vi "AlliGator Source Image Profile Window.vi"() -> ()   [LabVIEW 2021, in "AlliGator Image Profile Window.lvlib"]
doc: "AlliGator Profile Window."
uses:
  AlliGator Image Profile Window.lvlib
  Globals, Variables, Constants/AlliGator Variables List.ctl
  Action Engine/AlliGator Q Element.ctl
  Action Engine/AlliGator Q Event.ctl
  AlliGator Image Profile Data.ctl
  Image/Image ROI Type.ctl
  AlliGator Image Profile Plot Data.ctl
  Graphs/XY Graph/XY Plot Data.ctl
  Graphs/XY Graph/XY Graph Event.ctl
  <vilib>/Utility/miscctls.llb/LVPoint32TypeDef.ctl
  Image/Box Profile Type.ctl
  Graphs/XY Graph/XY Graph Add-Ons.lvlib
  Globals, Variables, Constants/AlliGator Globals, Variables & Constants.lvlib
  Notebook/Notebook.lvlib
  Rich Text Box/Rich Text Box.lvlib
  Settings/AlliGator Settings.lvlib
  Image/Image.lvlib
  Action Engine/AlliGator Action Engine.lvlib
  Error/Error.lvlib
panel:
  out "Image Profile TipStrip":string
  out "Image Profile":cluster{"X Array":dbl[], "Y Array":dbl[]}[](graph) caption="No Selection Profile (0,0)-(0,0)"
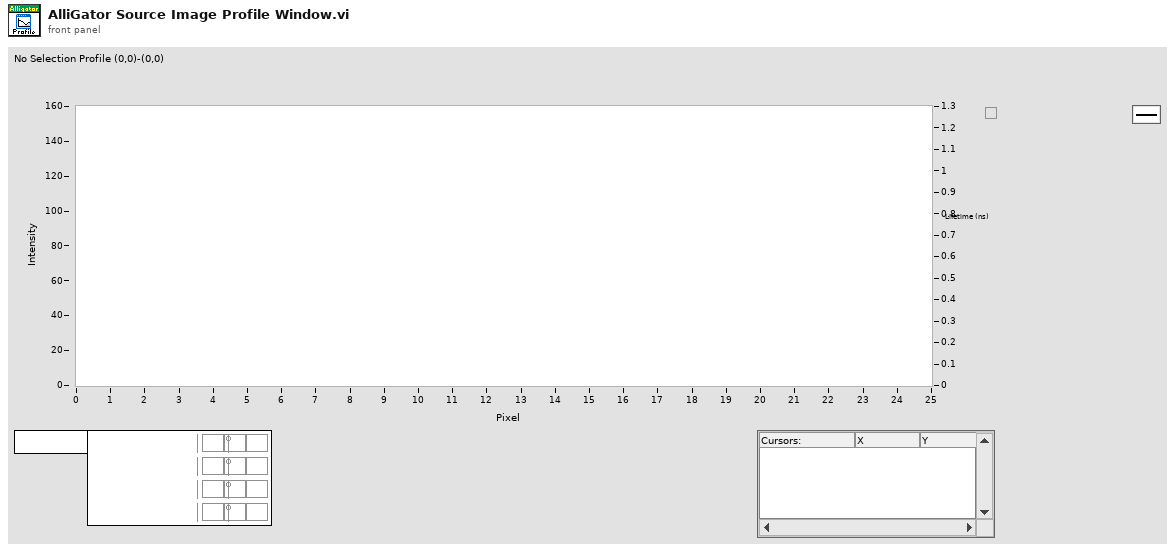
[diagram p1: front panel]
types:
  T1 = typedef "AlliGator Action Engine.lvlib/AlliGator Q Element.ctl" = cluster{"AlliGator Q Event":T2, "Data":variant}
  T2 = typedef "AlliGator Action Engine.lvlib/AlliGator Q Event.ctl" = enum16{"---- Files ----", "Files:Set Batch Export Files To Save", "Files:Set Dataset Loading & Pre-processing Options", "Files:Check #Frames in Dataset", "Files:Increment Frame Index", "Files:Open Mask Image", "Files:Open White Light Image", "Files:Open Single Dataset", "Files:New Folder of Folders Selected", "Files:Load File (all Types)_Scriptable", "Files:Move Flattened Series to Folders Series", "Files:Select Folder", "Files:Load FLI Dataset", "Files:Load Swiss SPAD 1 Dataset", "Files:Load Swiss SPAD 2 Dataset", "Files:Load .sdt FLI Dataset", "Files:Load .ptu FLI Dataset", "Files:Load .bin FLI Dataset", "Files:Load Single Gate Image Folder", "Files:Load I/m/phi Dataset (deprecated)", "Files:Load Single Image", "Files:Subtract Background File", "Files:Export FLI Dataset", "Files:Load HDF5 FLI Dataset", "Files:Set Destination File Path", "Files:Save Mask Image", "Files:Batch Conversion", "Files:New Folder Selected", "Files:Close FLI Dataset", "Files:Close FLI Dataset Series", "Files:Close White Light Image", "Files:Close Mask Image", "---- FLI Dataset ----", "FLI Dataset:Channel Arithmetic", "FLI Dataset:Export Average Lifetime Map as ASCII", "FLI Dataset:Export User-Defined Quantity Map as ASCII", "FLI Dataset:Python Function FLI Dataset Event", "FLI Dataset:ROI Analysis", "FLI Dataset:Tilted Logistic Square Gated IRF Characteristics Map", "FLI Dataset:Logistic Square Gated IRF Characteristics Map", "FLI Dataset:Square Gated IRF Characteristics Map", "FLI Dataset:Multi-ROI Single-Pixel Phasor Analysis", "FLI Dataset:Multi-ROI Single-Pixel NLSF Analysis", "FLI Dataset:All ROIs IRF Extraction", "FLI Dataset:All ROIs Decay Fit Non-Interactive (Fast + Individual IRF)", "FLI Dataset:All ROIs Phasor Analysis", "FLI Dataset:All ROIs Decay Fit", "FLI Dataset:Fluorescence Decay Statistics", "FLI Dataset:Update Decay Statistics Graph", "FLI Dataset:Get Decay from ROI", "FLI Dataset:All ROIs Average Lifetimes", "FLI Dataset:Save/Load Local IRFs", "FLI Dataset:Clear Local IRFs", "---- FLI Dataset Series ----", "FLI Dataset Series:Sum All Datasets in Series", "FLI Dataset Series:Add Dataset to Accumulated Dataset", "FLI Dataset Series:Display Accumulated Dataset", "FLI Dataset Series:Clear Dataset Series Sum", "FLI Dataset Series:Time-Series Analysis (NLSF)", "FLI Dataset Series:Time-Series Analysis (Phasor)", "---- Image ----", "Image:Update Image Profile Plots", "Image:Image Histogram Cursor Move", "Image:Image Histogram", "Image:Image Contrast", "Image:Set Image Histogram Cursor Move Flag", "Image:Clear Image Overlay", "Image:Use ROI as Search Area", "Image:Set ROI Diameter", "Image:Save Image Data as TIFF", "Image:Save Displayed Image with Overlay", "Image:Save Image Overlay Only", "Image:Save Image as Hot Pixel Mask", "Image:Change Source Image Color Palette", "Image:Copy Image to Clipboard", "Image:Source Image ROI Selection", "Image:Delete All ROIs", "Image:Delete All Unselected ROIs", "Image:Delete ROI", "Image:Merge All ROIs", "Image:Store ROI", "Image:Source Image ROI Storage", "Image:Export ROI Description to Notebook", "Image:Save ROI", "Image:Load ROI", "Image:Paste ROI Definition", "Image:Clear ROI", "Image:Identify ROIs in Mask Image", "Image:Create Complementary ROI", "Image:Create Contour ROI", "Image:Create ROI(s) from Pixels with Peak above Min_Scriptable", "Image:Create ROI(s) from Pixels with Intensity above Min_Scriptable", "Image:Compute ROI Statistics", "Image:Delete ROI(s) based on ROI Characteristics", "Image:Create ROI Grid", "Image:ROI to Individual Pixel ROIs", "Image:Python Function Source Image Event", "Image:Show Phasor Calibration Map ROI Centers", "Image:Convert ROI to Mask Image", "Image:Mouse Move", "Image:Mouse Up", "Image:Set Source Image Mouse Move Flag", "Image:Add Scale Bar Overlay", "Image:Delete Existing ROIs Option", "Image:Overlay ROI Median", "Image:Check Current ROI", "---- Decay ----", "Decay:Clear IRF/Reference Plot", "Decay:Add Decay to Graph", "Decay:Smoothen Plot", "Decay:Smoothen Plot Tail", "Decay:Average Selected Plots", "Decay:Extract IRF", "Decay:Optimal IRF Extraction", "Decay:Threshold IRF", "Decay:Fit to Model IRF", "Decay:Fit IRF to Square Gate", "Decay:Fit IRF to Logistic Square Gate", "Decay:Fit IRF to Tilted Logistic Square Gate", "Decay:Create Bounding Cursors Set", "Decay:Export Bounding Cursors Definition to Notebook", "Decay:Denoise Plot", "Decay:Compute Cumulative Function", "Decay:Use as Reference Decay", "Decay:Show Reference Decay/IRF", "Decay:Extrapolate Decay", "Decay:Create Head & Tail Bounding Cursors", "Decay:Store Cursor-defined Head & Tail Fractions", "Decay:Rebin Plot", "Decay:1-Normalize Decay", "Decay:[0-1]-Normalize Plot", "Decay:Straighten Decay", "Decay:Shift Decay", "Decay:Fold Decay", "Decay:Fit Decay", "Decay:Global Fit of Selected Decays", "Decay:Post Global Fit Script", "Decay:Add Global Fit Parameters to Graph", "Decay:Add Decay Parameter(s) to Plot (Graph)", "Decay:Export Decay to Phasor Graph", "Decay:Plot Decay Shifts", "Decay:Compute Average Lifetime", "Decay:Plot Convolution", "Decay:Graph Tip Strip Update", "---- Decay Statistics ----", "Decay Statistics:Tip Strip Update", "---- Intensity Time Trace ----", "Intensity Time Trace:Use File Timestamp", "Intensity Time Trace:Load Intensity Corrections File", "Intensity Time Trace:Clear Intensity Corrections File", "Intensity Time Trace:Tip Strip Update", "---- Phasor Plot ----", "Phasor Plot:Build Phasor Plot", "Phasor Plot:Change Phasor Plot Color Palette", "Phasor Plot:Adjust Phasor Plot Display Range", "Phasor Plot:Highlight Image ROI in Phasor Plot", "Phasor Plot:Save Phasor Plot Image with Overlay", "Phasor Plot:Export Complex Phasor Map", "Phasor Plot:Export Phasor Ratio Map", "Phasor Plot:Export Average Lifetime Map", "Phasor Plot:Compute Phase Lifetime Histogram", "Phasor Plot:Compute Phasor Ratio Histogram", "Phasor Plot:Compute Phase Lifetime vs Intensity Scatter Plot", "Phasor Plot:Weber 2-Component Decomposition", "Phasor Plot:Update Phasor Color Map Vertices", "Phasor Plot:Clear Phasor Overlay", "Phasor Plot:Use Segment Extremities as References", "Phasor Plot:Use UC/Segment Intersections as References", "Phasor Plot:Use UC/Principal Axis Intersections as References", "Phasor Plot:Use UC/Linear Fit Intersections as References", "Phasor Plot:Update Phasor Plot Reference", "Phasor Plot:Show Local Phasor Info in Phasor Plot", "Phasor Plot:Update Phasor Plot State", "Phasor Plot:Phasor Plot ROI Storage", "Phasor Plot:Phasor Plot ROI Selection", "Phasor Plot:Python Function Phasor Plot Event", "Phasor Plot:Overlay Phasor ROI, Ratio or Map in Source Image", "Phasor Plot:Compute Decay of Selected Phasors", "Phasor Plot:Phasor at Image Pixel", "Phasor Plot:Mouse Move", "Phasor Plot:Mouse Up", "Phasor Plot:Display Range Mouse Move", "Phasor Plot:Set Mouse Move Flag", "---- Phasor Graph ----", "Phasor Graph:Calibrated Phasor Map Series", "Phasor Graph:Whole Image Phasor Scatter Plot (deprecated)", "Phasor Graph:Get Phasor Value", "Phasor Graph:Create New Phasor Plot Dialog", "Phasor Graph:Update Last Phasor Value", "Phasor Graph:Update Phasor (m, phi)", "Phasor Graph:Remove Single Phasor from Plot", "Phasor Graph:Add Single Phasor to Plot", "Phasor Graph:Remove Phasor Plot", "Phasor Graph:Remove Selected Phasor Plots", "Phasor Graph:Clear Phasor Data", "Phasor Graph:Clear Phasor Graph", "Phasor Graph:Cursor Move", "Phasor Graph:Draw Cursor Connecting Line", "Phasor Graph:Clear Cursor Connecting Line", "Phasor Graph:Find UC Intersection", "Phasor Graph:Use UC/Cursor-Defined Line Intersections", "Phasor Graph:Use Selected Plots Fitted Line/UC Intersections", "Phasor Graph:Use Selected Plots Principal Axis/UC Intersections", "Phasor Graph:Show Single Phasor", "Phasor Graph:Save Single Phasor Plot", "Phasor Graph:Save All Phasor Plots", "Phasor Graph:Load Phasor Plot(s)", "Phasor Graph:Phasor Multiplication", "Phasor Graph:Compute Average Phasor", "Phasor Graph:Compute Multiple Average Phasors (Selected Plots)", "Phasor Graph:Export Single Phasor Plot Phase Lifetimes", "Phasor Graph:Phase Lifetime Trajectory (deprecated)", "Phasor Graph:Phase Lifetime vs Intensity Scatter Plot (deprecated)", "Phasor Graph:Parameter 2 vs Parameter 1 Scatter Plot", "Phasor Graph:Use Cursor n Location", "Phasor Graph:Set Reference n to Current Phase Lifetime Value", "Phasor Graph:Set Reference n to Lifetime Value", "Phasor Graph:Set Cursor n Location", "Phasor Graph:Save Phasor Graph Image", "Phasor Graph:Update SEPL Plot", "Phasor Graph:Export Single Phasor Plot Data", "Phasor Graph:Export Selected Phasor Plots Data", "Phasor Graph:Python Function Phasor Graph Event", "Phasor Graph:Tip Strip Update", "---- Calibration ----", "Calibration:Set Calibration Type", "Calibration:Load/Save Phasor Calibration", "Calibration:Load/Save Phasor Calibration Series", "Calibration:Load/Save Phasor Calibration Map", "Calibration:Use as Calibration", "Calibration:Compute Optimal Calibration from Phasor References", "Calibration:Clear Phasor Calibration", "Calibration:Single Phasor Calibration Information", "Calibration:Use as Calibration Series", "Calibration:Use as Calibration Map", "Calibration:Clear Calibration Series", "Calibration:Phasor Calibration Series Information", "Calibration:Clear Calibration Map", "Calibration:Phasor Calibration Map Information", "Calibration:Apply Phasor Calibration", "Calibration:Update Single Plot Calibration", "Calibration:Update Multiple Plots Calibration", "Calibration:Clear Single Plot Calibration", "Calibration:Clear All Plots Calibrations", "Calibration:Clear Plot(s) Calibration(s)?", "Calibration:Phasor Calibration Maps (# Gates Series)", "---- Phasor Ratio ----", "Phasor Ratio:Clear Reference n", "Phasor Ratio:Toggle Selected Plot(s)  Lock to Reference 1", "Phasor Ratio:Use as Reference n", "Phasor Ratio:Send Reference n to Notebook", "Phasor Ratio:Toggle Selected Plot(s)  Lock to Reference 2", "Phasor Ratio:Compute Phasor Ratio at Mouse Location", "Phasor Ratio:Compute Phasor Plot's Average Phasor Ratio", "Phasor Ratio:Compute Time-Series Phasor Ratios", "Phasor Ratio:Fit Line to Phasor Ratio Plot", "Phasor Ratio:Save References", "Phasor Ratio:Load References", "Phasor Ratio:Update Phasor Reference 1", "Phasor Ratio:Update Phasor Reference 2", "Phasor Ratio:Move Cursor n to Reference n", "Phasor Ratio:Use as Phasor Reference 1 Lifetime", "Phasor Ratio:Use as Phasor Reference 2 Lifetime", "Phasor Ratio:Export Phasor Ratio Map as ASCII", "Phasor Ratio:Tip Strip Update", "---- Lifetime & Other Parameters Graph ----", "Lifetime:Power Law from Intensity Distribution", "---- Decay Fit Parameter Map ----", "Decay Fit Parameter Map:Export ROI NLSF Data as ASCII", "Decay Fit Parameter Map:Set Decay Fit Parameter Map Selection", "Decay Fit Parameter Map:Build Decay Fit Parameter Map", "Decay Fit Parameter Map:Change Decay Fit Parameter Map Color Palette", "Decay Fit Parameter Map:Export Decay Fit Parameter Map Data as ASCII", "Decay Fit Parameter Map:Export All Decay Fit Parameter Maps Data as ASCII", "Decay Fit Parameter Map:Selected Parameter Scatterplot", "Decay Fit Parameter Map:Parameter 2 vs Parameter 1 Scatterplot", "Decay Fit Parameter Map:Save Decay Fit Parameter Map Image", "Decay Fit Parameter Map:Save-Load IRFs & Fit Data", "Decay Fit Parameter Map:Update Local Decay Plots", "Decay Fit Parameter Map:Python Function Decay Fit Parameters Map Event", "Decay Fit Parameter Map:Overlay Decay Fit Parameter Map in Source Image", "Decay Fit Parameter Map:Selected Parameter vs Intensity Scatterplot", "Decay Fit Parameter Map:Mouse Up", "Decay Fit Parameter Map:Display Range Mouse Move", "Decay Fit Parameter Map:Change Map Resolution", "---- Parameter Map ----", "Parameter Map:Export ROI Parameters Data as ASCII", "Parameter Map:Delete Parameter Map Set", "Parameter Map:Update Parameter List", "Parameter Map:Build Parameter Map", "Parameter Map:Change Parameter Map Color Palette", "Parameter Map:Export Parameter Map Data as ASCII", "Parameter Map:Export All Parameter Maps Data as ASCII", "Parameter Map:Selected Parameter Scatterplot", "Parameter Map:Parameter 2 vs Parameter 1 Scatterplot", "Parameter Map:Selected Parameter vs Intensity Scatterplot", "Parameter Map:Save Parameter Map Image", "Parameter Map:Save-Load IRFs & Parameter Maps (TODO)", "Parameter Map:Set Parameter Map Selection", "Parameter Map:Python Function Parameter Map Event", "Parameter Map:Overlay Parameter Map in Source Image", "Parameter Map:Update Local Decay Plots", "Parameter Map:Mouse Up", "Parameter Map:Display Range Mouse Move", "---- Generic Graph ----", "Generic Graph:Generic XY Graph Event", "Generic Graph:Python Function XY Graph Event", "Generic Graph:New Plot", "Generic Graph:Save Plot", "Generic Graph:XY Plot Histogram", "Generic Graph:Set XY Graph Plot Name", "Generic Graph:Set Last Cursor Style", "Generic Graph:Tip Strip Update", "---- GUI ----", "GUI:Start Script", "GUI:Type of Displayed Image Changed", "GUI:Gate Image Slide Changed", "GUI:Show Busy Icon", "GUI:Show Busy Icon & Abort Button", "GUI:Hide Busy Icon", "GUI:Hide Busy Icon & Abort Button", "GUI:Abort", "GUI:End Script", "GUI:Start Timing", "GUI:End Timing", "GUI:Set State Indicator", "GUI:Send Parameters JSON Strings to Clipboard", "GUI:Set Gate Step", "GUI:Idle", "GUI:Initialization", "GUI:Quit", "GUI:Increment Dataset Index", "GUI:Set Dataset Index to -1", "GUI:Time Series Slider Moved", "GUI:Time Series Slider Changed", "GUI:Toggle Playback or Loop", "GUI:Playback Script", "GUI:Set Phasor Frequency", "GUI:Open Window", "GUI:Start Test Script", "GUI:End Test Script", "DEBUG"}
  T3 = typedef "AlliGator Globals, Variables & Constants.lvlib/AlliGator Variables List.ctl" = enum16{"---- GUI ----", "GUI:Initialization Status", "GUI:State Indicators Refnum", "GUI:Original AlliGator Menu Items", "GUI:Current Action Loop State", "GUI:Script in progress", "GUI:Playback", "GUI:Loop Playback", "GUI:Search ROI Used", "GUI:Search ROI", "Decay Graph Max Legend Size", "Intensity Graph Max Legend Size", "Decay Statistics Graph Max Legend Size", "Phasor Graph Max Legend Size", "Phasor Ratio Graph Max Legend Size", "Lifetime Graph Max Legend Size", "---- Files ----", "Files:Export Dataset Frames as Individual Files", "Files:Show Batch Export Help Balloons", "Files:Frames in Dataset", "Files:ptu File Frame Start Indices", "Files:Current Frame in Dataset", "Files:Current Frame Timestamp", "Files:Dataset Loaded", "Files:Dataset Metadata", "Files:Dataset Channel", "Files:Dataset Data Description", "Files:Background Dataset Metadata", "Files:Background Dataset Channel", "Files:Background Dataset Data Description", "Files:Background File Subtraction", "Files:Background File Path", "Files:Background File Pile-up Correction", "Files:Background File Pixel Well Capacity", "Files:Background File Scaling Factor", "Files:Current Dataset Load Settings", "Files:Dataset Path", "Files:ICCD-specific Information", "Files:Macrotime Gate Separation", "------ Python Plugins ------", "Python Plugins:Information", "Python Plugins:Python Session", "Python Plugins:Valid Python Session?", "---- Source Image ----", "Source Image:ROIs", "Source Image:Current ROI", "Source Image:ROI Event Refnum", "X_Source Image:Display Range", "X_Source Image:Palette Information", "X_Source Image:Type of Displayed Image", "X_Time Gate Slider", "Source Image:Palette List", "Source Image:Scale", "Source Image:ROI Overlay Color", "Source Image:Overlay to Erase", "Source Image:Is Displayed Image Accumulated", "Source Image:White Light Image Modified", "Source Image:Mask Image Modified", "---- Image Profile Window ----", "Image Profile:Window Event Refnum", "Image Profile:IntensityType", "Image Profile:Intensity Average Type", "Image Profile:Intensity-weighted SDV", "Image Profile:Box Profile Type", "Image Profile:Window Open", "Image Profile:Plotted Fit Parameter", "------ Phasor Graph -------", "Phasor Graph:Show Line", "---- Phasor Plot ---", "Phasor Plot:Parameters Changed", "Phasor Plot:FLI Dataset Modified since last Calculation", "Phasor Harmonics Data", "Selected Phasor Harmonics", "Phasor Harmonic Manager Event Refnum", "Phasor Plot:ROIs", "Phasor Plot:Current ROI", "Phasor Plot:ROI Event Refnum", "Phasor Plot:Image Reference Points", "Phasor Plot:Computed", "Phasor Plot:Palette Information", "Phasor Plot:Palette List", "Phasor Plot:Phasor Ratio Palette Information", "Phasor Plot:Phasor Ratio Palette List", "Phasor Plot:Image Scale", "Phasor Plot:Image Overlay to Erase", "Phasor Plot:Image Elements to Update", "Phasor Plot:Current Calculation Parameters", "Phasor Plot:Current Calibration Options", "Phasor Plot:Reset Cumulated Phasor Plot", "Phasor Plot:Reference 1", "Phasor Plot:Lifetime Reference 1", "Phasor Plot:Reference 1 Frequency", "Phasor Plot:Reference 2", "Phasor Plot:Lifetime Reference 2", "Phasor Plot:Reference 2 Frequency", "---- Decay Analysis ----", "Number of Selected Decays to Fit", "LS Fit Results", "LAR Fit Results", "BS Fit Results", "Last Decay Max - Min", "Best Fit Parameters", "Best Fit Parameter Names", "Actual Size X", "Actual Size Y", "Binning X", "Binning Y", "Actual # Gates", "Dataset Number", "Gates to...", "Gates Skipped", "Gates to keep", "Gate Step", "Gate Separation", "Reversed Gates", "Pile-up Correction", "Pixel Well Capacity", "Background Subtracted", "Background Subtraction Method", "Background Definition Range", "Background File (deprecated)", "Number of Dataset Accumulated", "Array of Accumulated Dataset Paths", "Do Averaged Datasets", "Destination File Path", "Process Plot Target", "Use 1/D as Phasor Frequency", "---- Decay Fit Parameter Map -----", "Decay Fit Parameter Map:Palette Information", "Decay Fit Parameter Map:Palette List", "Decay Fit Parameter Map:X Resolution", "Decay Fit Parameter Map:Y Resolution", "---- Parameter Map ----", "Parameter Map:Palette Information", "Parameter Map:Palette List", "------- Local Decay Window ---------", "Local Decay Graph Window:Event Refnum", "Local Decay Graph Window:Use normalized IRF for convolution", "----- Miscellaneous ----", "Misc:Skippable Dialog Windows Status"}
  T4 = enum32{"Invalid", "Standard", "Closed", "Hidden", "Minimized", "Maximized"}
  T5 = typedef "XY Graph Add-Ons.lvlib/XY Graph Refnum.ctl" = refnum<vi>
  T6 = cluster{"Event Registration Refnum":refnum<event-registration>, "Event Registration Refnum":refnum<event-registration>}
  T7 = typedef "XY Graph Add-Ons.lvlib/XY Graph Event.ctl" = cluster{"Item Tag":string, "XY Graph Refnum":refnum<vi>, "Coords":T8, "Item Path":string}
  T8 = typedef "LVPoint32TypeDef.ctl" = cluster{"Horizontal":i32, "Vertical":i32}
  T9 = typedef "Image.lvlib/Box Profile Type.ctl" = enum16{"Full Width", "Half Width"}
  T10 = typedef "Rich Text Box.lvlib/Text Formatting.ctl" = cluster{"Font":string, "Text Color":T11, "Text Background Color":T11, "Text Style":enum16{"Regular", "Bold", "Italic", "Underline", "Strikeout"}, "Font Size (Points)":dbl, "Text Alignment":i32}
  T11 = typedef "Rich Text Box.lvlib/Text Colors.ctl" = enum16{"Unchanged", "Black", "Blue", "Brown", "Gray", "Green", "Orange", "Pink", "Red", "White"}
  T12 = typedef "AlliGator Image Profile Window.lvlib/AlliGator Image Profile Plot Data.ctl" = cluster{"Plot Name":string, "Plot":T13}
  T13 = typedef "XY Graph Add-Ons.lvlib/XY Plot Data.ctl" = cluster{"X Array":dbl[], "Y Array":dbl[]}
  T14 = typedef "Image.lvlib/Image ROI Type.ctl" = enum16{"No Selection", "Point", "Line", "Rectangle", "Oval", "Polygon", "Freehand Region", "Annulus", "Unused2", "Unused3", "Broken Line", "Freehand Line", "Rotated Rectangle"}
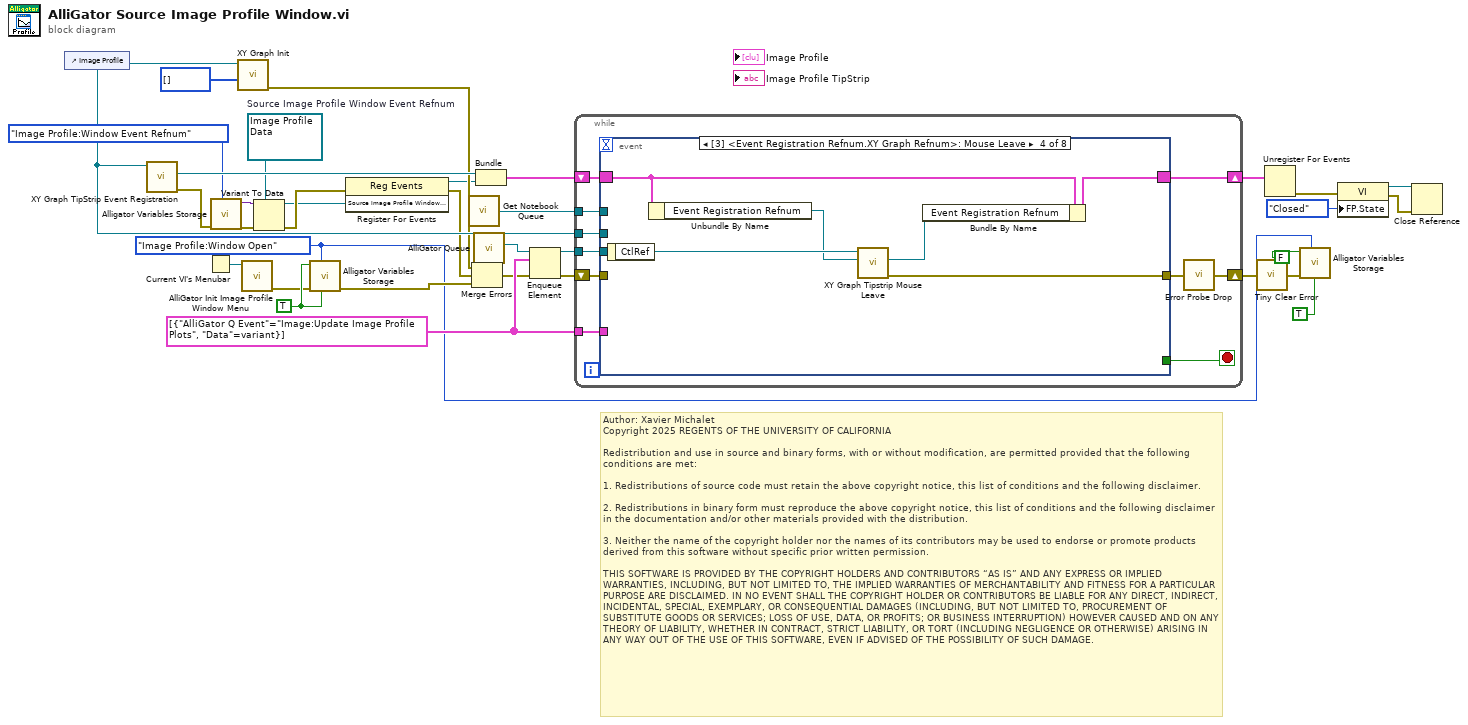
[diagram p0: block diagram]
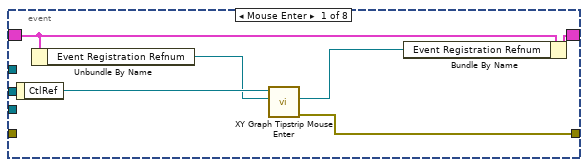
[diagram p2: hidden frame]
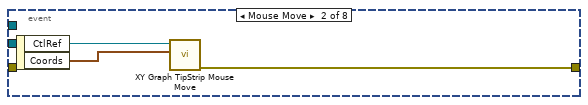
[diagram p3: hidden frame]
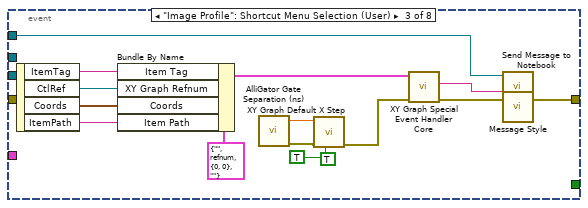
[diagram p4: hidden frame]
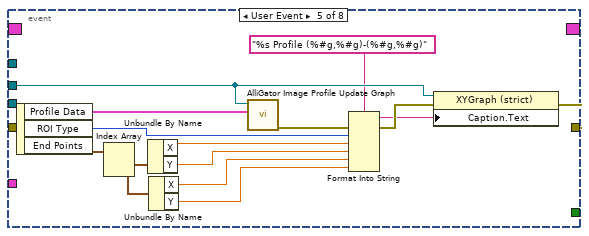
[diagram p5: hidden frame]
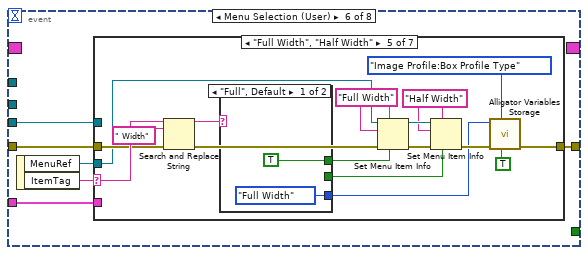
[diagram p6: hidden frame]
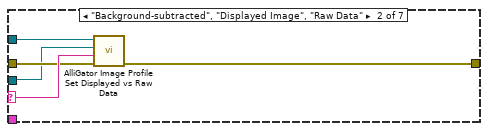
[diagram p8: hidden frame]
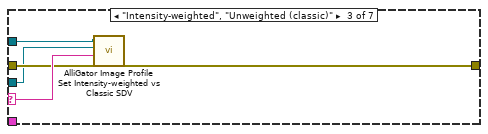
[diagram p9: hidden frame]
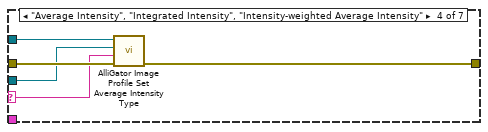
[diagram p10: hidden frame]
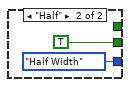
[diagram p11: hidden frame]
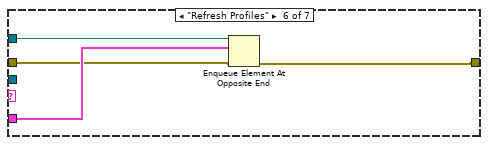
[diagram p12: hidden frame]
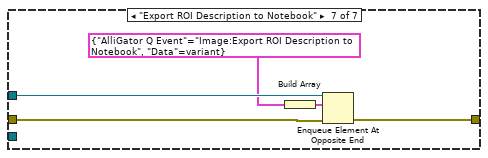
[diagram p13: hidden frame]
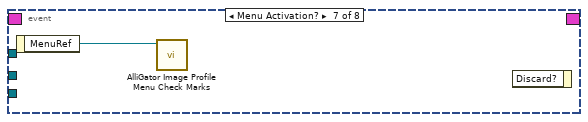
[diagram p14: hidden frame]
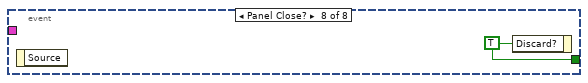
[diagram p15: hidden frame]
diagram:
  w3 = refnum<user-event> refnum  # Source Image Profile Window Event Refnum
  w7 = T1[] [{"AlliGator Q Event"=enum."Image:Update Image Profile Plots", "Data"=variant}] ("element")
  w14 = TRUE (".not. x?")
  w4 = AlliGator_Variables_List."Image Profile:Window Open" ("Alligator Variable")
  # "Author: Xavier Michalet\nCopyright 2025 REGENTS OF THE UNIVERSITY OF CALIFORNIA\n\nRedistribution and use in source and binary forms, with or without modification, are permitted provided that the following conditions are met:\n\n1. Redistributions of source code must retain the above copyright notice, this list of conditions and the following disclaimer.\n\n2. Redistributions in binary form must reproduce the above copyright notice, this list of conditions and the following disclaimer in the documentation and/or other materials provided with the distribution.\n\n3. Neither the name of the copyright holder nor the names of its contributors may be used to endorse or promote products derived from this software without specific prior written permission.\n\nTHIS SOFTWARE IS PROVIDED BY THE COPYRIGHT HOLDERS AND CONTRIBUTORS “AS IS” AND ANY EXPRESS OR IMPLIED WARRANTIES, INCLUDING, BUT NOT LIMITED TO, THE IMPLIED WARRANTIES OF MERCHANTABILITY AND FITNESS FOR A PARTICULAR PURPOSE ARE DISCLAIMED. IN NO EVENT SHALL THE COPYRIGHT HOLDER OR CONTRIBUTORS BE LIABLE FOR ANY DIRECT, INDIRECT, INCIDENTAL, SPECIAL, EXEMPLARY, OR CONSEQUENTIAL DAMAGES (INCLUDING, BUT NOT LIMITED TO, PROCUREMENT OF SUBSTITUTE GOODS OR SERVICES; LOSS OF USE, DATA, OR PROFITS; OR BUSINESS INTERRUPTION) HOWEVER CAUSED AND ON ANY THEORY OF LIABILITY, WHETHER IN CONTRACT, STRICT LIABILITY, OR TORT (INCLUDING NEGLIGENCE OR OTHERWISE) ARISING IN ANY WAY OUT OF THE USE OF THIS SOFTWARE, EVEN IF ADVISED OF THE POSSIBILITY OF SUCH DAMAGE."
  n1 = control-ref of="Image Profile"() -> (w27:refnum<vi>)
  n2 = call "XY Graph TipStrip Event Registration.vi"("XY Graph Refnum"=w27) -> ("error out"=w18:errorcluster, "Event Registration Refnum"=w33:refnum<event-registration>, "XY Graph Refnum"=w28:T5)  [unwired: 8 in]
  n3 = Current VI's Menubar() -> (w12:refnum<k9>)
  n4 = call "Alligator Variables Storage.vi"("AlliGator Variable"=AlliGator_Variables_List."Image Profile:Window Event Refnum" ("Alligator Variable"), "Error In"=w18) -> ("Error Out"=w24:errorcluster, "Data out"=w25:variant)  [unwired: 7 in, 1 out]
  n5 = call "XY Graph Init.vi"("Plots to Skip (none)"=i32[] [], "XYGraph in"=w28) -> ("Error Out"=w17:errorcluster)  [unwired: 9 in]
  n6 = call "AlliGator Init Image Profile Window Menu.vi"("Menu in"=w12) -> ("error out"=w11:errorcluster)  [unwired: 10 in]
  n7 = Variant To Data(error in=w24, type=w3, Variant=w25) -> (data=w22:refnum<user-event>, error out=w23:errorcluster)
  n8 = call "Alligator Variables Storage.vi"("Get(F)/Set"=w14, "AlliGator Variable"=w4, "Error In"=w11, "Data in"=w14) -> ("Error Out"=w16:errorcluster)  [unwired: 5 in, 2 out]
  n9 = register-events(error in=w23, w22) -> (reference out=w2:refnum<event-registration>, error out=w19:errorcluster)  [unwired: 1 in]
  n10 = call "Get Notebook Queue.vi"() -> ("Notebook Queue"=w20:refnum<queue>)  [unwired: 9 in]
  n11 = Merge Errors(w17, w19, w16) -> (w5:errorcluster)
  n12 = call "AlliGator Queue.vi"() -> ("AlliGator Q"=w9:refnum<queue>)  [unwired: 8 in, 1 out]
  n13 = Bundle("Event Registration Refnum"=w33, "Event Registration Refnum"=w2) -> (w21:T6)  [unwired: 1 in]
  n14 = Enqueue Element(queue=w9, element=w7, error in (no error)=w5) -> (queue out=w8:refnum<queue>, error out=w6:errorcluster)  [unwired: 1 in, 1 out]
  n15 = while {
    shift-right: [w44] -> w34
    shift-left: w21 -> [w45]
    tunnel: w27 -> [w43]
    tunnel: w20 -> [w42]
    shift-right: [w36] -> w15
    shift-left: w6 -> [w39]
    tunnel: w8 -> [w38]
    tunnel: w7 -> [w37]
    stop <- w40 stop-if-true
    n16 = event shown="[3] <Event Registration Refnum.XY Graph Refnum>: Mouse Leave" {
      selector: w45 -> [w49 _ _ w72 _ _ _ _]
      dyn-events: [w51 _ _ w71 _ _ _ _] -> w44
      timeout: _ -> [_ _ _ _ _ _ _ _]
      tunnel: [_ _ _ _ _ _ _ w144] -> w40
      tunnel: w43 -> [_ _ _ _ w89 _ _ _]
      tunnel: w42 -> [_ _ w67 _ _ _ _ _]
      tunnel: [w46 w52 w65 w70 w88 w94 _ _] -> w41
      tunnel: w39 -> [_ _ _ _ _ w93 _ _]
      tunnel: w38 -> [_ _ _ _ _ w92 _ _]
      tunnel: w37 -> [_ _ _ _ _ w91 _ _]
      event Mouse Enter {
        n17 = event-data() -> ("CtlRef"=w50:refnum<vi>)  [unwired: 1 in]
        n18 = Unbundle By Name(w49) -> ("Event Registration Refnum"=w48:refnum<event-registration>)
        n19 = call "XY Graph Tipstrip Mouse Enter.vi"("Event Registration Refnum"=w48, "XY Graph Refnum"=w50) -> ("Error Out"=w46:errorcluster, "Event Registration Refnum"=w47:refnum<event-registration>)  [unwired: 8 in]
        n20 = Bundle By Name(cluster=w49, "Event Registration Refnum"=w47) -> (w51:T6)
      }
      event Mouse Move {
        n21 = event-data() -> ("CtlRef"=w54:refnum<vi>, "Coords"=w53:T8)  [unwired: 1 in]
        n22 = call "XY Graph TipStrip Mouse Move.vi"("Coords"=w53, "XY Graph Refnum"=w54) -> ("Error Out"=w52:errorcluster)  [unwired: 7 in, 2 out]
      }
      event "Image Profile": Shortcut Menu Selection (User) {
        (unwired) TRUE ("Get (F)/Set")
        n23 = event-data() -> ("ItemTag"=w64:string, "CtlRef"=w63:refnum<vi>, "Coords"=w62:T8, "ItemPath"=w61:string)  [unwired: 1 in]
        n24 = Bundle By Name(cluster=T7 {"Item Tag"="", "XY Graph Refnum"=refnum, "Coords"={"Horizontal"=0, "Vertical"=0}, "Item Path"=""} ("XY Graph Event"), "Item Tag"=w64, "XY Graph Refnum"=w63, "Coords"=w62, "Item Path"=w61) -> (w59:T7)
        n25 = call "AlliGator Gate Separation (ns).vi"() -> ("error out"=w58:errorcluster, "Gate Separation (ns)"=w56:dbl)  [unwired: 10 in]
        n26 = call "XY Graph Default X Step.vi"("Get (F)/Set"=TRUE, "Error In"=w58, "Default X Step"=w56) -> ("Error Out"=w57:errorcluster)  [unwired: 7 in, 1 out]
        n27 = call "XY Graph Special Event Handler Core.vi"("error in (no error)"=w57, "XY Graph Event"=w59) -> ("error out"=w69:errorcluster, "Message"=w68:string)  [unwired: 5 in, 3 out]
        n28 = call "Message Style.vi"() -> ("Message Formatting"=w66:T10)
        n29 = call "Send Message to Notebook.vi"("Text Formatting"=w66, "Error In"=w69, "Message"=w68, "Notebook Queue"=w67) -> ("Error Out"=w65:errorcluster)  [unwired: 4 in, 1 out]
      }
      event Mouse Leave {
        n30 = event-data() -> ("CtlRef"=w75:refnum<vi>)  [unwired: 1 in]
        n31 = Unbundle By Name(w72) -> ("Event Registration Refnum"=w74:refnum<event-registration>)
        n32 = call "XY Graph Tipstrip Mouse Leave.vi"("Event Registration Refnum"=w74, "XY Graph Refnum"=w75) -> ("Error Out"=w70:errorcluster, "Event Registration Refnum"=w73:refnum<event-registration>)  [unwired: 8 in]
        n33 = Bundle By Name(cluster=w72, "Event Registration Refnum"=w73) -> (w71:T6)
      }
      event User Event {
        n34 = event-data() -> ("Profile Data"=w90:T12[], "ROI Type"=w84:T14, "End Points"=w82:cluster{"X":dbl, "Y":dbl}[])  [unwired: 1 in]
        n35 = Index Array(array=w82) -> (element #1=w81:cluster{"X":dbl, "Y":dbl}, element #2=w78:cluster{"X":dbl, "Y":dbl})  [unwired: 2 in]
        n36 = Unbundle By Name(w81) -> ("X"=w80:dbl, "Y"=w79:dbl)
        n37 = Unbundle By Name(w78) -> ("X"=w77:dbl, "Y"=w76:dbl)
        n38 = call "AlliGator Image Profile Update Graph.vi"("Profile Data"=w90, "XY Graph Refnum"=w89) -> ("Error Out"=w87:errorcluster)  [unwired: 9 in]
        n39 = Format Into String(format string="%s Profile (%#g,%#g)-(%#g,%#g)", error in=w87, w84, w80, w79, w77, w76) -> (resulting string=w85:string, error out=w86:errorcluster)  [unwired: 1 in]
        n40 = property class="XYGraph (strict)"(reference=w89, error in=w86, "Caption.Text"=w85) -> (error out=w88:errorcluster)  [unwired: 1 out]
      }
      event Menu Selection (User) {
        n41 = event-data() -> ("MenuRef"=w96:refnum<k9>, "ItemTag"=w95:string)  [unwired: 1 in]
        n42 = case shown="\"Full Width\", \"Half Width\"" w95 {
          selector: w95 -> [_ w102 w107 w109 w129 _ _]
          tunnel: w96 -> [_ w99 w104 w108 w113 _ _]
          tunnel: [w97 w101 w106 w110 w117 w135 w140] -> w94
          tunnel: w93 -> [w97 w100 w105 w111 w120 w134 w141]
          tunnel: w92 -> [_ w98 w103 w112 _ w137 w142]
          tunnel: w91 -> [_ _ _ _ _ w136 _]
          frame "", Default {
          }
          frame "Background-subtracted", "Displayed Image", "Raw Data" {
            n43 = call "AlliGator Image Profile Set Displayed vs Raw Data.vi"("Error In"=w100, "ItemTag"=w102, "Menu in"=w99, "AlliGator Queue"=w98) -> ("Error Out"=w101:errorcluster)  [unwired: 7 in]
          }
          frame "Intensity-weighted", "Unweighted (classic)" {
            n44 = call "AlliGator Image Profile Set Intensity-weighted vs Classic SDV.vi"("Error In"=w105, "ItemTag"=w107, "Menu in"=w104, "AlliGator Queue"=w103) -> ("Error Out"=w106:errorcluster)  [unwired: 7 in]
          }
          frame "Average Intensity", "Integrated Intensity", "Intensity-weighted Average Intensity" {
            n45 = call "AlliGator Image Profile Set Average Intensity Type.vi"("Error In"=w111, "ItemTag"=w109, "Menu in"=w108, "AlliGator Queue"=w112) -> ("Error Out"=w110:errorcluster)  [unwired: 7 in]
          }
          frame "Full Width", "Half Width" {
            w122 = "Half Width" ("item tag")
            w123 = "Full Width" ("item tag")
            n46 = Search and Replace String(input string=w129, search string=" Width", error in=w120) -> (result string=w127:string, error out=w119:errorcluster)  [unwired: 5 in, 2 out]
            n47 = case shown="\"Full\", Default" w127 {
              tunnel: [TRUE ("checked") _] -> w126
              tunnel: [_ TRUE ("checked")] -> w124
              tunnel: [Box_Profile_Type."Full Width" Box_Profile_Type."Half Width"] -> w116
              frame "Full", Default {
              }
              frame "Half" {
              }
            }
            n48 = Set Menu Item Info(6:w126, 7:w123, 8:w119, 10:w123, 11:w113) -> (0:w121:errorcluster, 3:w125:refnum<k9>)  [unwired: 2 in]
            n49 = Set Menu Item Info(6:w124, 7:w122, 8:w121, 10:w122, 11:w125) -> (0:w118:errorcluster)  [unwired: 2 in, 1 out]
            n50 = call "Alligator Variables Storage.vi"("Get(F)/Set"=TRUE, "AlliGator Variable"=AlliGator_Variables_List."Image Profile:Box Profile Type" ("Alligator Variable"), "Error In"=w118, "Data in"=w116) -> ("Error Out"=w117:errorcluster)  [unwired: 5 in, 2 out]
          }
          frame "Refresh Profiles" {
            n51 = Enqueue Element At Opposite End(queue=w137, element=w136, error in (no error)=w134) -> (error out=w135:errorcluster)  [unwired: 1 in, 2 out]
          }
          frame "Export ROI Description to Notebook" {
            n52 = Build Array(T1 {"AlliGator Q Event"=enum."Image:Export ROI Description to Notebook", "Data"=variant} ("Time-Gated Phasor Q Element")) -> (w139:T1[])
            n53 = Enqueue Element At Opposite End(queue=w142, element=w139, error in (no error)=w141) -> (error out=w140:errorcluster)  [unwired: 1 in, 2 out]
          }
        }
      }
      event Menu Activation? {
        n54 = event-data() -> ("MenuRef"=w143:refnum<k9>)  [unwired: 1 in]
        n55 = call "AlliGator Image Profile Menu Check Marks.vi"("Menu in"=w143) -> ()  [unwired: 10 in, 1 out]
        n56 = event-data() -> ()  [unwired: 2 in, 1 out]
      }
      event Panel Close? {
        w144 = TRUE ("Discard?")
        n57 = event-data() -> ()  [unwired: 1 in, 1 out]
        n58 = event-data("Discard?"=w144) -> ()  [unwired: 1 in, 1 out]
      }
    }
    n59 = call "Error Probe Drop.vi"("error in (no error)"=w41) -> ("error out"=w36:errorcluster)
  }
  n60 = call "Tiny Clear Error.vi"("Error In"=w15) -> ("no Error Out"=w1:errorcluster)  [unwired: 8 in]
  n61 = Unregister For Events(event registration refnum=w34) -> (error out=w32:errorcluster)  [unwired: 1 in]
  n62 = call "Alligator Variables Storage.vi"("Get(F)/Set"=TRUE (".not. x?"), "AlliGator Variable"=w4, "Error In"=w1, "Data in"=FALSE (".not. x?")) -> ()  [unwired: 5 in, 3 out]
  n63 = property class="VI"(error in=w32, "FP.State"=T4."Closed" ("Front Panel Window:State")) -> (reference out=w30:refnum<vi>, error out=w29:errorcluster)  [unwired: 1 in]
  n64 = Close Reference(reference=w30, error in (no error)=w29) -> ()  [unwired: 1 out]
